vi "control main.vi"() -> ()   [LabVIEW 2013]
uses:
  <vilib>/userdefined/High Color/IMAQdx.ctl
  <vilib>/vision/driver/NI_Vision_Acquisition_Software.lvlib
panel:
  out "CAMERA":T1(plugin-control)
  in  "Session In":T2
  in  "stop 3":bool
  in  "Tab Control":enum32{"control ", " IMU data"}(tab)
  in  "stop":bool
  out "forward":bool
  out "right":bool
  out "backword":bool
  out "left":bool
  in  "throtel":dbl(knob) scale=0.0..180.0
  out "RPM":dbl(knob) scale=0.0..180.0
  out "temperature":dbl(slide) scale=0.0..100.0
  in  "milliseconds to wait 4":u32
  in  "stop 2":bool
  out "Z 2":i16
  out "Y 2":i16
  out "X 2":i16
  in  "milliseconds to wait 2":u32
  in  "stop 4":bool
  out "?":dbl
  in  "milliseconds to wait":u32
  in  "stop 5":bool
  out "Y":i16
  out "Z":i16
  out "X":i16
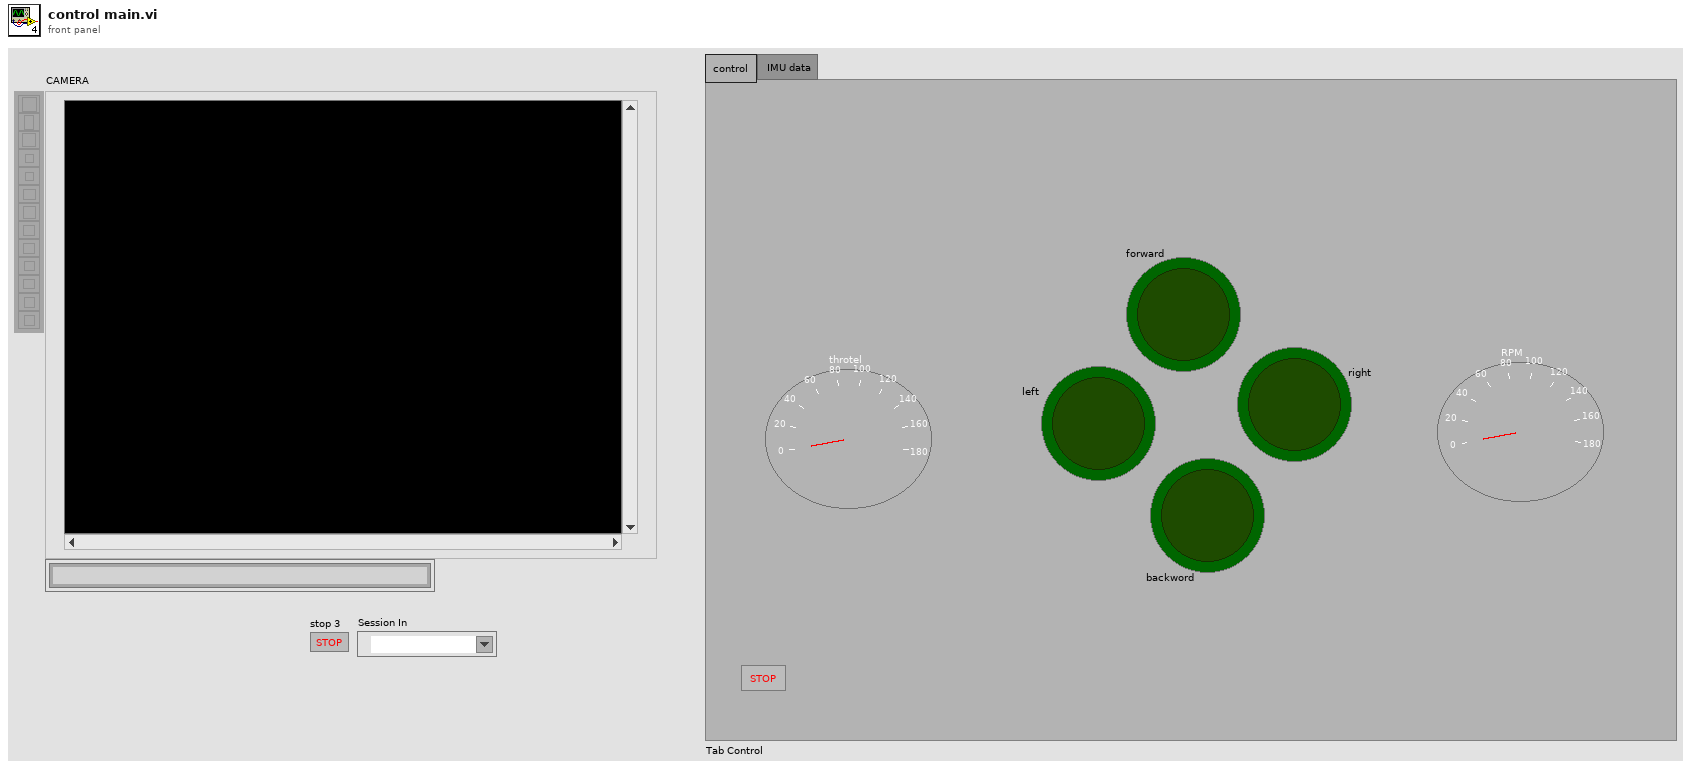
[diagram p1: front panel]
types:
  T1 = typedef "IMAQ Image.ctl" = refnum<image>
  T2 = typedef "IMAQdx.ctl" = refnum<k21>
  T3 = typedef "Image Type" = u32
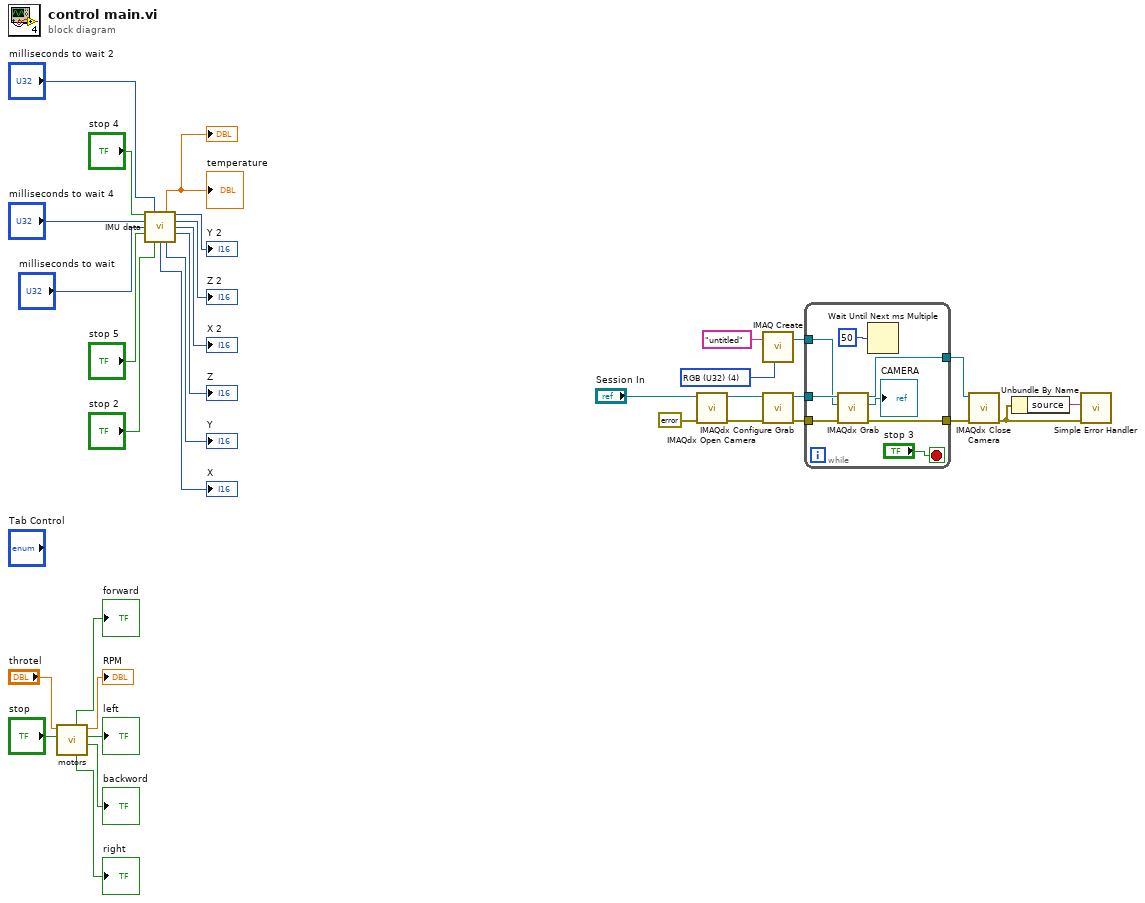
[diagram p0: block diagram]
diagram:
  w4 = T3 4 items=["Grayscale (U8)", "Grayscale (I16)", "Grayscale (SGL)", "Complex (CSG)", "RGB (U32)", "HSL (U32)", "RGB (U64)", "Grayscale (U16)"] ("Image Type")
  n1 = call "motors.vi"("stop"="stop", "throtel"="throtel") -> ("backword"=→"backword":bool, "left"=→"left":bool, "RPM"=→"RPM":dbl, "right"=→"right":bool, "forward"=→"forward":bool)  [unwired: 5 in]
  n2 = call "IMU data.vi"("stop 4"="stop 4", "milliseconds to wait 2"="milliseconds to wait 2", "milliseconds to wait 4"="milliseconds to wait 4", "milliseconds to wait"="milliseconds to wait", "stop 5"="stop 5", "stop in"="stop 2") -> (3:→"?" →"temperature":dbl, "Y 2"=→"Y 2":i16, "Z 2"=→"Z 2":i16, "X 2"=→"X 2":i16, "Z"=→"Z":i16, "X"=→"X":i16, "Y"=→"Y":i16)  [unwired: 3 in]
  n3 = call <vilib>:"IMAQdx Open Camera.vi"("error in"=errorcluster {"status"=FALSE, "code"=0, "source"=""}, "Session In"="Session In") -> ("error out"=w8:errorcluster, "Session Out"=w9:T2)  [unwired: 8 in]
  n4 = call "IMAQ Create"("Image Name"="untitled", "Image Type"=w4) -> ("New Image"=w3:T1)  [unwired: 3 in, 1 out]
  n5 = call <vilib>:"IMAQdx Configure Grab.vi"("error in"=w8, "Session In"=w9) -> ("error out"=w7:errorcluster, "Session Out"=w6:T2)  [unwired: 8 in]
  n6 = while {
    tunnel: w6 -> [w40]
    tunnel: w7 -> [w39]
    tunnel: [w38] -> w11
    tunnel: [w37] -> w10
    tunnel: w3 -> [w36]
    stop <- "stop 3" stop-if-true
    n7 = call <vilib>:"IMAQdx Grab.vi"("error in"=w39, "Image In"=w36, "Session In"=w40) -> ("error out"=w38:errorcluster, "Image Out"=→"CAMERA":T1, "Session Out"=w37:T2)  [unwired: 5 in, 1 out]
    n8 = Wait Until Next ms Multiple(millisecond multiple=u32 50) -> ()  [unwired: 1 out]
  }
  n9 = call <vilib>:"IMAQdx Close Camera.vi"("error in"=w11, "Session In"=w10) -> ("error out"=w2:errorcluster)  [unwired: 9 in]
  n10 = Unbundle By Name(w2) -> ("source"=w1:string)
  n11 = call <vilib>:"Simple Error Handler.vi"("error source (\" \")"=w1, "error in (no error)"=w2) -> ()  [unwired: 3 in, 5 out]
